vi "subHamamatsu_OpenCam.vi"(5 "Exposure (ms)":dbl=100.0 caption="Exposure (msec)" min=1.0 max=5000.0 step=1.0, 7 "ROI":T2={"Bin"=2, "ROI"={"x offset"=256, "y offset"=256, "x width"=512, "y width"=512}} {"ROI"."x offset" min=1 max=512 step=1; "ROI"."y offset" min=1 max=512 step=1; "ROI"."x width" min=1 max=512 step=1; "ROI"."y width" min=1 max=512 step=1; "Bin" items=["1x1"=1, "2x2"=2, "4x4"=4]}, 8 "error in (no error)":errorcluster {"code" format="%.0x"}, 10 "Camera Setting":T3={"Camera Output triger mode setiting"={"Mode"=3, "Polarity"=2, "Period"=0.0005, "Delay"=0.0}, "Camera timing port for trigering"=enum."3"} {"Camera Output triger mode setiting"."Polarity" items=["Negative"=1, "Positive"=2]; "Camera Output triger mode setiting"."Mode" items=["Low"=1, "Global Exposure"=2, "Programmable"=3, "Trigger Ready"=4, "High"=5]}, 11 "Handle in":u32) -> (0 "error out":errorcluster, 2 "Camera in use":T1={"Model"="", "Camera ID"="", "Bits"=16}, 3 "Handle out":u32)   [LabVIEW 2015]
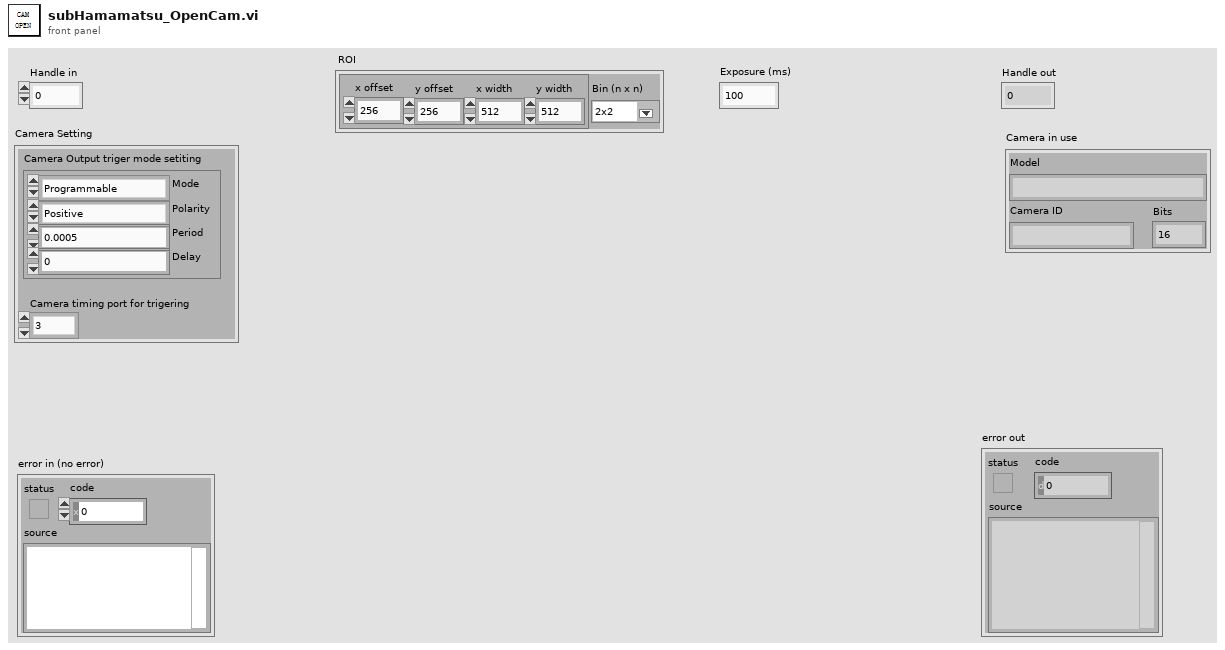
[diagram p1: front panel]
types:
  T1 = cluster{"Model":string, "Camera ID":string, "Bits":i32}
  T2 = cluster{"Bin":u16, "ROI":cluster{"x offset":i32, "y offset":i32, "x width":i32, "y width":i32}}
  T3 = cluster{"Camera Output triger mode setiting":cluster{"Mode":u32, "Polarity":u32, "Period":dbl, "Delay":dbl}, "Camera timing port for trigering":enum16{"1", "2", "3"}}
  T4 = cluster{"Mode":u32, "Polarity":u32, "Period":dbl, "Delay":dbl}
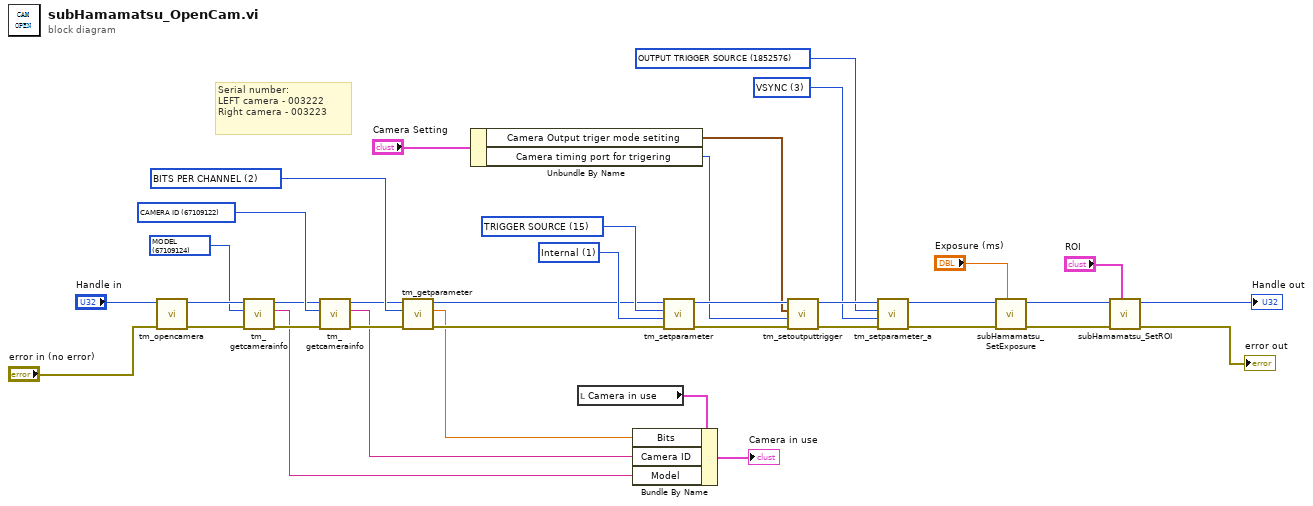
[diagram p0: block diagram]
diagram:
  w16 = u16 3 items=["READOUT END"=2, "VSYNC"=3]
  w20 = u32 1852576 items=["SENSOR MODE"=4212128, "CCD MODE"=4212384, "READOUT MODE"=4211872, "ACTIVE VIEW INDEX"=4343136, "BITS PER CHANNEL"=4342976, "IMAGE PIXEL TYPE"=4343296, "BINNING"=4215968, "EXPOSURE TIME"=2049184, "CONTRAST GAIN"=3163312, "CONTRAST OFFSET"=3163328, "LIGHT MODE"=2114720, "SENSITIVITY"=2114992, "PHOTON IMAGING MODE"=2115200, "HIGH DYNAMIC RANGE MODE"=3163360, "WHITE BALANCE"=3163568, "TEMPERATURE"=2115232, "TEMPERATURE TARGET"=2115264, "SENSOR COOLER FAN"=2115296, "LINEBUNDLE HEIGHT"=4212192, "MECHANICAL SHUTTER"=2115488, "BACK FOCUS POSITION"=8422304, "TRIGGER CONNECTOR"=1066432, "TRIGGER SOURCE"=1066144, "OUTPUT TRIGGER SOURCE"=1852576, "TRIGGER GLOBAL EXPOSURE"=2049680, "FIRST TRIGGER BEHAVIOR"=2049696, "CHANNEL SYNC"=1852352, "READOUT DIRECTION"=4211904, "PRE HSYNC COUNT"=1852704, "INTERNAL LINE SPEED"=4226000, "INTERNAL LINE INTERVAL"=4226016] ("Parameter")
  w31 = 2 items=["BINNING"=1, "BITS PER CHANNEL"=2, "ACTIVE VIEW INDEX"=3, "CCD MODE"=4, "SENSOR MODE"=5, "READOUT MODE"=6, "EXPOSURE TIME"=7, "CONTRAST GAIN"=8, "CONTRAST OFFSET"=9, "LIGHT MODE"=10, "SENSITIVITY"=11, "WHITE BALANCE"=12, "PHOTON IMAGING MODE"=13, "HIGH DYNAMIC RANGE MODE"=14, "TRIGGER SOURCE"=15, "TRIGGER ACTIVE"=16, "TRIGGER MODE"=17, "TRIGGER POLARITY"=18, "TRIGGER GLOBAL EXPOSURE"=19, "FIRST TRIGGER BEHAVIOR"=20, "TRIGGER TIMES"=21, "OUTPUT TRIGGER POLARITY"=22, "OUTPUT TRIGGER DELAY"=23, "OUTPUT TRIGGER PERIOD"=24, "TEMPERATURE"=25, "TEMPERATURE TARGET"=26, "SENSOR COOLER FAN"=27, "MECHANICAL SHUTTER"=28, "BACK FOCUS POSITION"=29, "FRAMEBUNDLE MODE"=30, "FRAMEBUNDLE NUMBER"=31, "LINEBUNDLE HEIGHT"=32, "TRIGGER CONNECTOR"=33, "IMAGE PIXEL TYPE"=34] ("Parameter")
  w28 = u32 67109122 items=["BUS"=67109121, "CAMERA ID"=67109122, "VENDOR"=67109123, "MODEL"=67109124, "CAMERA VERSION"=67109125, "DRIVER VERSION"=67109126, "MODULE VERSIOIN"=67109127, "DCAMAPI VERSION"=67109128] ("Info ID")
  w29 = u32 67109124 items=["BUS"=67109121, "CAMERA ID"=67109122, "VENDOR"=67109123, "MODEL"=67109124, "CAMERA VERSION"=67109125, "DRIVER VERSION"=67109126, "MODULE VERSIOIN"=67109127, "DCAMAPI VERSION"=67109128] ("Info ID")
  w37 = 1 items=["Internal"=1, "External"=2, "Software"=3] ("Trigger Source")
  w36 = 15 items=["BINNING"=1, "BITS PER CHANNEL"=2, "ACTIVE VIEW INDEX"=3, "CCD MODE"=4, "SENSOR MODE"=5, "READOUT MODE"=6, "EXPOSURE TIME"=7, "CONTRAST GAIN"=8, "CONTRAST OFFSET"=9, "LIGHT MODE"=10, "SENSITIVITY"=11, "WHITE BALANCE"=12, "PHOTON IMAGING MODE"=13, "HIGH DYNAMIC RANGE MODE"=14, "TRIGGER SOURCE"=15, "TRIGGER ACTIVE"=16, "TRIGGER MODE"=17, "TRIGGER POLARITY"=18, "TRIGGER GLOBAL EXPOSURE"=19, "FIRST TRIGGER BEHAVIOR"=20, "TRIGGER TIMES"=21, "OUTPUT TRIGGER POLARITY"=22, "OUTPUT TRIGGER DELAY"=23, "OUTPUT TRIGGER PERIOD"=24, "TEMPERATURE"=25, "TEMPERATURE TARGET"=26, "SENSOR COOLER FAN"=27, "MECHANICAL SHUTTER"=28, "BACK FOCUS POSITION"=29, "FRAMEBUNDLE MODE"=30, "FRAMEBUNDLE NUMBER"=31, "LINEBUNDLE HEIGHT"=32, "TRIGGER CONNECTOR"=33, "IMAGE PIXEL TYPE"=34] ("Parameter")
  # "Serial number:\nLEFT camera - 003222\nRight camera - 003223"
  n1 = call "tm_opencamera.vi"("error in (no error)"="error in (no error)", "Camera Index"="Handle in") -> ("error out"=w27:errorcluster, "Handle out"=w33:u32)  [unwired: 8 in]
  n2 = call "tm_getcamerainfo.vi"("error in (no error)"=w27, "Info ID"=w29, "Handle in"=w33) -> ("error out"=w30:errorcluster, "String"=w13:string, "Handle out"=w26:u32)  [unwired: 6 in]
  n3 = call "tm_getcamerainfo.vi"("error in (no error)"=w30, "Info ID"=w28, "Handle in"=w26) -> ("error out"=w32:errorcluster, "String"=w12:string, "Handle out"=w25:u32)  [unwired: 6 in]
  n4 = call "tm_getparameter.vi"("error in (no error)"=w32, "Parameter"=w31, "Handle in"=w25) -> ("error out"=w35:errorcluster, "Value out"=w14:dbl, "Handle out"=w34:u32)  [unwired: 6 in]
  n5 = Unbundle By Name("Camera Setting") -> ("Camera Output triger mode setiting"=w4:T4, "Camera timing port for trigering"=w3:enum16{"1", "2", "3"})
  n6 = local read "Camera in use"() -> (w2:T1)
  n7 = Bundle By Name(cluster=w2, "Bits"=w14, "Camera ID"=w12, "Model"=w13) -> (→"Camera in use":T1)
  n8 = call "tm_setparameter.vi"("error in (no error)"=w35, "Value in"=w37, "Parameter"=w36, "Handle in"=w34) -> ("error out"=w17:errorcluster, "Handle out"=w18:u32)  [unwired: 6 in]
  n9 = call <userlib>:"tm_setoutputtrigger.vi"("error in (no error)"=w17, "Index"=w3, "Parameters"=w4, "Handle in"=w18) -> ("error out"=w22:errorcluster, "Handle out"=w21:u32)  [unwired: 6 in]
  n10 = call <userlib>:"tm_setparameter_a.vi"("error in (no error)"=w22, "Value in"=w16, "Parameter"=w20, "Handle in"=w21) -> ("error out"=w15:errorcluster, "Handle out"=w10:u32)  [unwired: 6 in]
  n11 = call "subHamamatsu_SetExposure.vi"("Exposure (ms)"="Exposure (ms)", "error in (no error)"=w15, "Handle in"=w10) -> ("error out"=w23:errorcluster, "Handle out"=w9:u32)  [unwired: 7 in]
  n12 = call "subHamamatsu_SetROI.vi"("ROI"="ROI", "error in (no error)"=w23, "Handle in"=w9) -> ("error out"=→"error out":errorcluster, "Handle out"=→"Handle out":u32)  [unwired: 6 in, 1 out]
